vi "LogForDuration.vi"(6 "Rate [Hz]":dbl=100.0, 7 "Log File Path (temporary file)":path, 8 "error in (no error)":errorcluster, 9 "milliseconds to wait":u32=1000, 10 "Channel Paths":string[](array[string]), 11 "VeriStand Test Case in":refnum<class "VeriStandTestCase.lvclass">) -> (0 "error out":errorcluster, 2 "data":waveform(dbl)[](array[waveform]), 3 "VeriStand Test Case out":refnum<class "VeriStandTestCase.lvclass">)   [LabVIEW 2015, in "VeriStandTestCase.lvclass"]
uses:
  VeriStandTestCase.lvclass
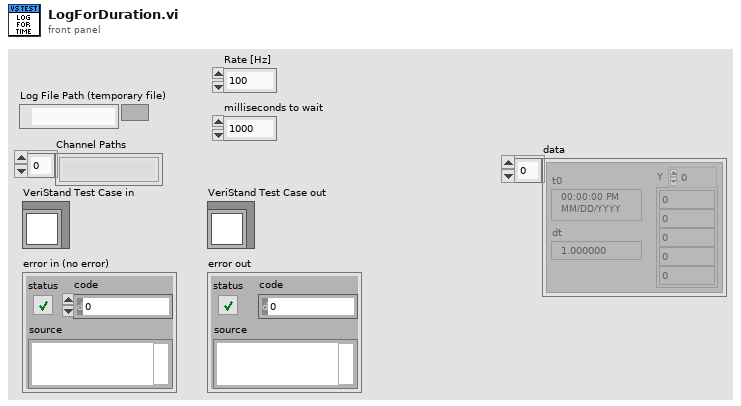
[diagram p1: front panel]
types:
  T1 = typedef "NI_VS Workspace ExecutionAPI.lvlib/LogFileConfiguration.ctl" = cluster{"File Path":path, "Description":string, "Trigger":T2, "Replace File":bool, "Rate [Hz]":dbl, "File Properties":T4[], "Channels":T5[]}
  T2 = typedef "NI_VS Workspace ExecutionAPI.lvlib/LogFileTriggerConfiguration.ctl" = cluster{"Type":T3, "Channel Path":string, "High Limit":dbl, "Low Limit":dbl}
  T3 = typedef "NI_VS Workspace ExecutionAPI.lvlib/LogFileTriggerType.ctl" = enum16{"None", "In Limits", "Out of Limits"}
  T4 = typedef "NI_VS Workspace ExecutionAPI.lvlib/LogProperty.ctl" = cluster{"Name":string, "Value":string}
  T5 = typedef "NI_VS Workspace ExecutionAPI.lvlib/LogChannelConfiguration.ctl" = cluster{"Channel Path":string, "Custom Name":string, "Custom Group":string, "Properties":T4[]}
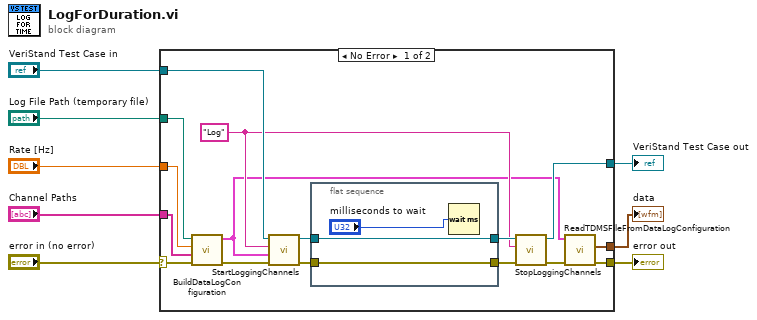
[diagram p0: block diagram]
diagram:
  n1 = case shown="No Error" "error in (no error)" {
    selector: "error in (no error)" -> [w11 w29]
    tunnel: [w24 w29] -> w8
    tunnel: [w23 w28] -> w7
    tunnel: [w22 _] -> w6
    tunnel: "Channel Paths" -> [w20 _]
    tunnel: "Log File Path (temporary file)" -> [w15 _]
    tunnel: "Rate [Hz]" -> [w14 _]
    tunnel: "VeriStand Test Case in" -> [w12 w28]
    frame No Error {
      w10 = "Log" ("Data Log Configuration Name")
      n2 = call "BuildDataLogConfiguration.vi"("error in (no error)"=w11, "Channel Paths"=w20, "Rate [Hz]"=w14, "Log File Path (temporary file)"=w15) -> ("error out"=w13:errorcluster, "Data Log File Configuration"=w9:T1)  [unwired: 6 in]
      n3 = call "StartLoggingChannels.vi"("error in (no error)"=w13, "Data Log File Configuration"=w9, "Data Log Configuration Name"=w10, "VeriStand Test Case in"=w12) -> ("error out"=w16:errorcluster, "VeriStand Test Case out"=w17:refnum<class "VeriStandTestCase.lvclass">)  [unwired: 6 in]
      n4 = flat-sequence {
        tunnel: w16 -> [w27]
        tunnel: [w27] -> w19
        tunnel: w17 -> [w26]
        tunnel: [w26] -> w18
        frame #0 {
          n5 = Wait (ms)(milliseconds to wait="milliseconds to wait") -> ()  [unwired: 1 out]
        }
      }
      n6 = call "StopLoggingChannels.vi"("error in (no error)"=w19, "Data Log Configuration Name"=w10, "VeriStand Test Case in"=w18) -> ("error out"=w21:errorcluster, "VeriStand Test Case out"=w23:refnum<class "VeriStandTestCase.lvclass">)  [unwired: 7 in]
      n7 = call "ReadTDMSFileFromDataLogConfiguration.vi"("error in (no error)"=w21, "Data Log File Configuration"=w9) -> ("error out"=w24:errorcluster, "data"=w22:waveform(dbl)[])  [unwired: 7 in, 1 out]
    }
    frame Error {
    }
  }
  "error out" <- w8
  "VeriStand Test Case out" <- w7
  "data" <- w6
